vi "pressure_transducer_transfer_func.vi"(1 "p_v":fxp<+/-,24,5>) -> (0 "pressure":fxp<+/-,32,16>)   [LabVIEW 2018]
uses:
  <vilib>/rvi/FXPMathLib/FxpMul/XNode/nifxpmath_Multiplier.xnode
  <vilib>/rvi/FXPMathLib/sim/FxpSim.dll
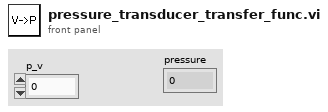
[diagram p1: front panel]
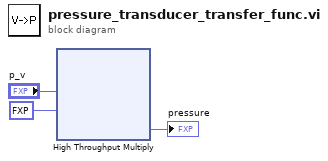
[diagram p0: block diagram]
diagram:
  n1 = xnode ("High Throughput Multiply")("x"="p_v", "y"=fxp<+,7,9> 300.0) -> ("x*y"=→"pressure":fxp<+/-,32,16>)
